vi "Directory to list File compare.vi"(6 "2nd File Type(s)(*.txt *.CSV)":string="*.zip", 7 "1st File Type(s)(*.txt *.CSV)":string="*.RAT", 8 "error in (no error)":errorcluster, 9 "2nd Directory (Zip)":path, 11 "1st Directory (RATS)":path) -> (0 "error out":errorcluster, 1 "Number of files Unmanaged":i32, 3 "Unmanaged Files":string[](array[string]))   [LabVIEW 2010]
doc: "Compare to see if there is a zip file for every rat file, if not then zip a copy and prep for FTP move"
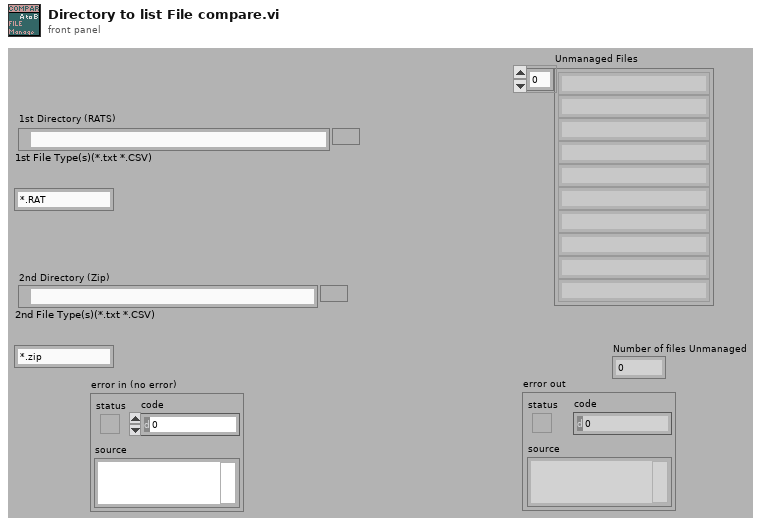
[diagram p1: front panel]
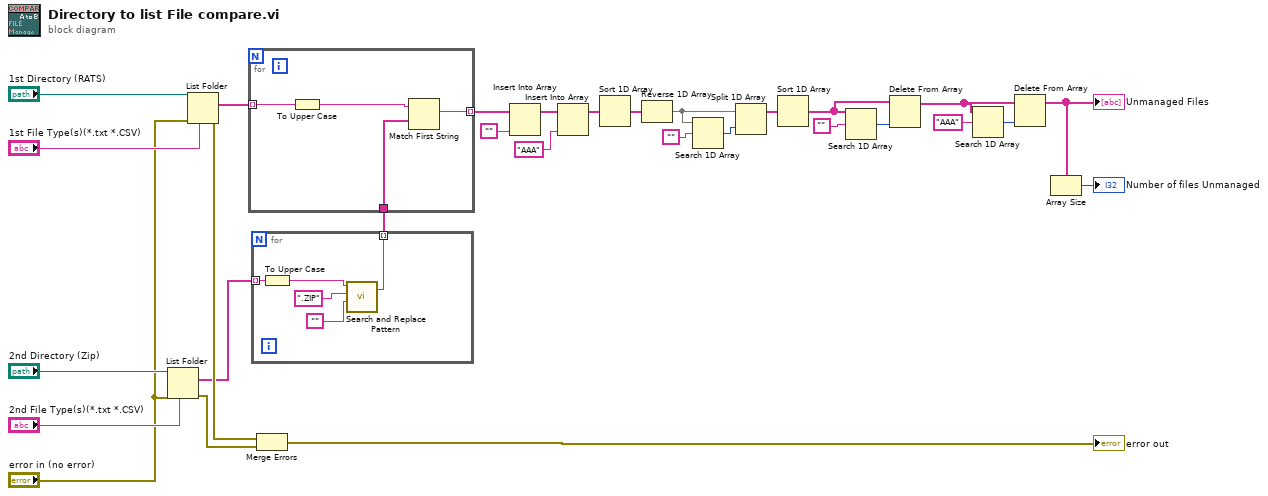
[diagram p0: block diagram]
diagram:
  n1 = List Folder(path="2nd Directory (Zip)", pattern="2nd File Type(s)(*.txt *.CSV)", error in="error in (no error)") -> (filenames=w3:string[], error out=w12:errorcluster)  [unwired: 1 in, 2 out]
  n2 = List Folder(path="1st Directory (RATS)", pattern="1st File Type(s)(*.txt *.CSV)", error in="error in (no error)") -> (filenames=w14:string[], error out=w13:errorcluster)  [unwired: 1 in, 2 out]
  n3 = for {
    tunnel: w3 -> [w31] mode=indexing
    tunnel: [w30] -> w2 mode=indexing
    n4 = To Upper Case(1:w31) -> (0:w34:string)
    n5 = call <vilib>:"Search and Replace Pattern.vi"("string"=w34, "regular expression (\"\")"=".ZIP" ("substring (\"\")"), "replace string (\"\")"="" ("replace string (\"\")")) -> ("result string"=w30:string)  [unwired: 2 in, 1 out]
  }
  n6 = for {
    tunnel: [w38] -> w21 mode=indexing
    tunnel: w14 -> [w36] mode=indexing
    tunnel: w2 -> [w37]
    n7 = To Upper Case(1:w36) -> (0:w35:string)
    n8 = Match First String(2:w37, 3:w35) -> (1:w38:string)  [unwired: 1 out]
  }
  n9 = Merge Errors(w13, w12) -> (→"error out":errorcluster)
  n10 = Insert Into Array(array=w21, new element="") -> (w23:string[])  [unwired: 1 in]
  n11 = Insert Into Array(array=w23, new element="AAA" ("new element/subarray")) -> (w20:string[])  [unwired: 1 in]
  n12 = Sort 1D Array(array=w20) -> (sorted array=w25:string[])
  n13 = Reverse 1D Array(array=w25) -> (reversed array=w24:string[])
  n14 = Search 1D Array(1D array=w24, element="") -> (index of element=w28:i32)  [unwired: 1 in]
  n15 = Split 1D Array(array=w24, index=w28) -> (first subarray=w19:string[])  [unwired: 1 out]
  n16 = Sort 1D Array(array=w19) -> (sorted array=w5:string[])
  n17 = Search 1D Array(1D array=w5, element="") -> (index of element=w9:i32)  [unwired: 1 in]
  n18 = Delete From Array(array=w5, index=w9) -> (array with subset deleted=w6:string[])  [unwired: 1 in, 1 out]
  n19 = Search 1D Array(1D array=w6, element="AAA" ("new element/subarray")) -> (index of element=w7:i32)  [unwired: 1 in]
  n20 = Delete From Array(array=w6, index=w7) -> (array with subset deleted=w4:string[])  [unwired: 1 in, 1 out]
  "Unmanaged Files" <- w4
  n21 = Array Size(array=w4) -> (size(s)=→"Number of files Unmanaged":i32)
